vi "GT Set Capture Offset.vi"(6 "loop":i32, 7 "count":i16, 8 "error in (no error)":errorcluster caption="错误输入（无错误）", 9 "pOffset":i32, 10 "encoder":i16, 11 "cardNum":i16) -> (0 "error out":errorcluster caption="错误输出", 1 "pOffset out":i32, 3 "function return":i16)   [LabVIEW 2020, in "gts1.lvlib"]
doc: "GT_API GT_SetCaptureOffset(short cardNum,short encoder,long *pOffset,short count=1,long loop=1);"
uses:
  gts1.lvlib
  dll/32bit/multi_card/gts.dll
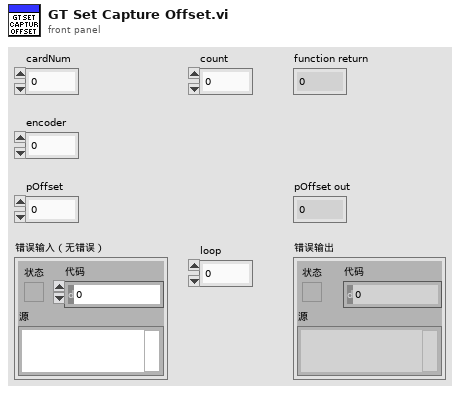
[diagram p1: front panel]
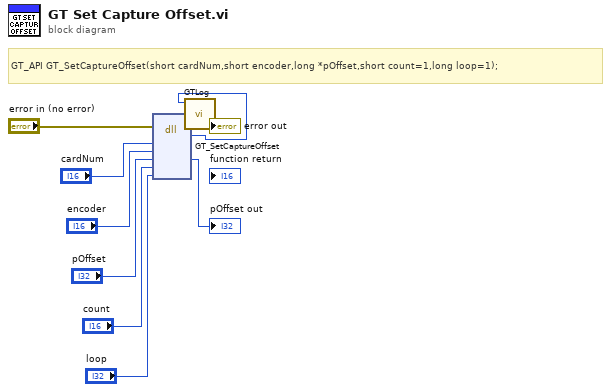
[diagram p0: block diagram]
diagram:
  # "GT_API GT_SetCaptureOffset(short cardNum,short encoder,long *pOffset,short count=1,long loop=1);"
  n1 = dll-call lib="C:/1228/dll/32bit/multi_card/gts.dll" fn="GT_SetCaptureOffset"(error in="error in (no error)", "cardNum"="cardNum", "encoder"="encoder", "pOffset"="pOffset", "count"="count", "loop"="loop") -> (error out=w3:errorcluster, w1:i16, "pOffset"=→"pOffset out":i32)  [unwired: 6 in, 1 out]
  n2 = call "GTLog.vi"("error in (no error)"=w3, "Numeric"=w1) -> ("error out"=→"error out":errorcluster)  [unwired: 9 in]
